vi "TotalPointsAuto.vi"(6 "Did they move?":string, 9 "Was the goal lit?":string, 11 "input":dbl) -> (3 "Total Auto Points":string)   [LabVIEW 2013]
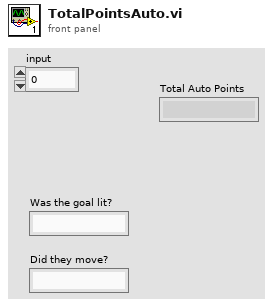
[diagram p1: front panel]
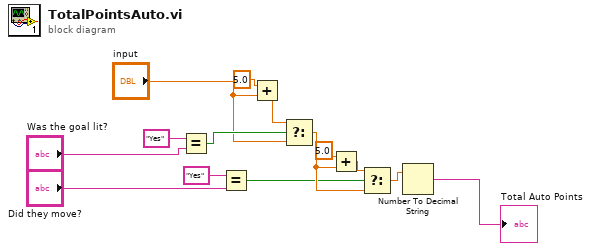
[diagram p0: block diagram]
diagram:
  n1 = Equal?(x="Yes", y="Was the goal lit?") -> (x = y?=w3:bool)
  n2 = Equal?(x="Yes", y="Did they move?") -> (x = y?=w7:bool)
  n3 = Add(x=5.0, y="input") -> (x+y=w5:dbl)
  n4 = Select(t=w5, s=w3, f="input") -> (s? t:f=w9:dbl)
  n5 = Add(x=5.0, y=w9) -> (x+y=w10:dbl)
  n6 = Select(t=w10, s=w7, f=w9) -> (s? t:f=w11:dbl)
  n7 = Number To Decimal String(number=w11) -> (decimal integer string=→"Total Auto Points":string)  [unwired: 1 in]
